vi "Calculate Saccade Gain.vi"(6 "Gain Window":T1, 7 "Impulse Data":refnum<data-value>, 8 "error in (no error)":errorcluster, 9 "Sample Rate (Hz)":dbl, 10 "Valid Range Fraction":dbl=1.0 format="%#_13g", 11 "Saccades in":T2[](array[typedef])) -> (0 "error out":errorcluster, 3 "Saccade out":T2[](array[typedef]))   [LabVIEW 2016]
uses:
  Saccade Analyser Saccade Data.ctl
  Saccade Analyser Impulse Data.ctl
  <vilib>/Analysis/NI_AALBase.lvlib
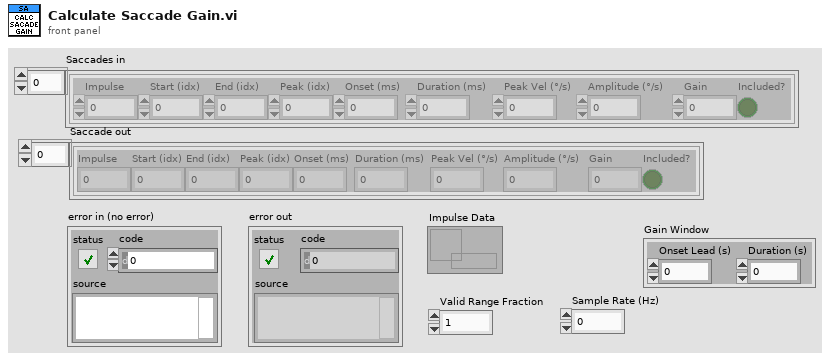
[diagram p1: front panel]
types:
  T1 = cluster{"Onset Lead (s)":dbl, "Duration (s)":dbl}
  T2 = typedef "Saccade Analyser Saccade Data.ctl" = cluster{"Impulse":i32, "Start (idx)":dbl, "End (idx)":dbl, "Peak (idx)":dbl, "Onset (ms)":dbl, "Duration (ms)":dbl, "Peak Vel (°/s)":dbl, "Amplitude (°/s)":dbl, "Gain":dbl, "Included?":bool}
  T3 = typedef "Saccade Analyser Impulse Data.ctl" = cluster{"Stimulus Data":dbl[], "Response Data":dbl[], "Peak (idx)":i32, "Onset (idx)":i32}
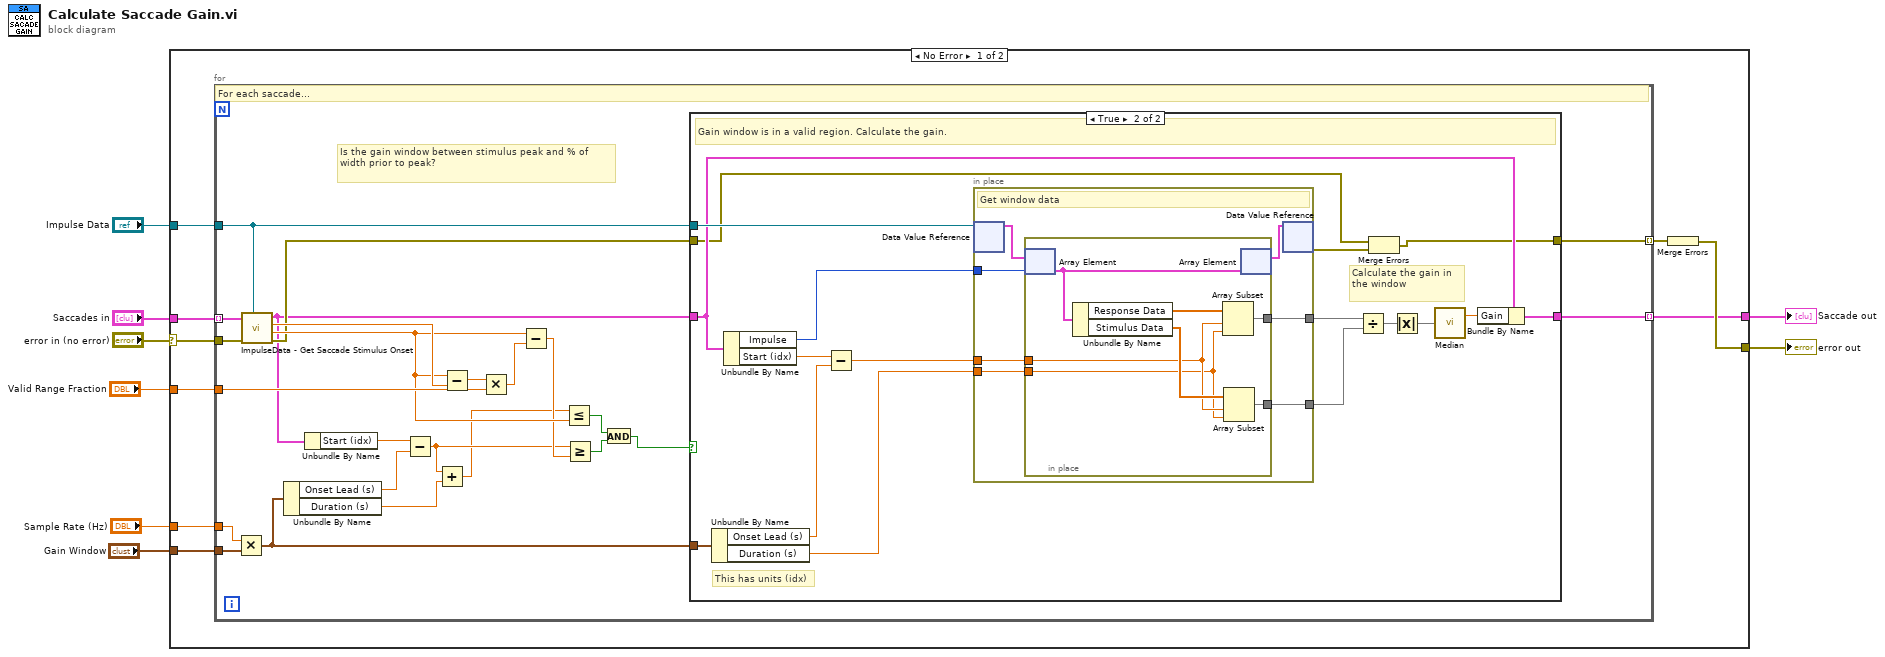
[diagram p0: block diagram]
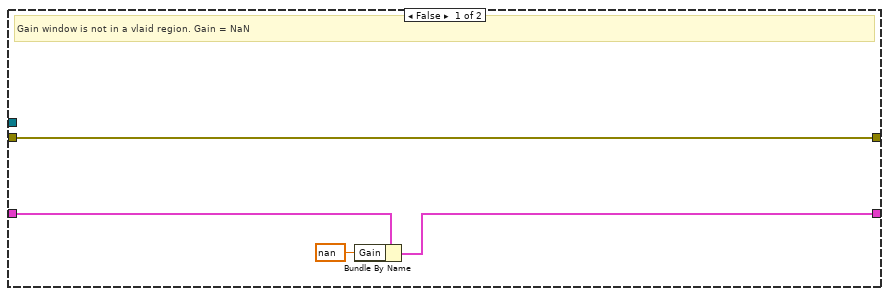
[diagram p2: hidden frame]
diagram:
  n1 = case shown="No Error" "error in (no error)" {
    selector: "error in (no error)" -> [w15 w77]
    tunnel: "Saccades in" -> [w17 w78]
    tunnel: [w12 w78] -> w5
    tunnel: [w14 w77] -> w7
    tunnel: "Impulse Data" -> [w16 _]
    tunnel: "Sample Rate (Hz)" -> [w13 _]
    tunnel: "Gain Window" -> [w11 _]
    tunnel: "Valid Range Fraction" -> [w10 _]
    frame No Error {
      n2 = for {
        tunnel: w17 -> [w38] mode=indexing
        tunnel: w16 -> [w36]
        tunnel: w15 -> [w37]
        tunnel: w13 -> [w40]
        tunnel: [w39] -> w12 mode=indexing
        tunnel: w11 -> [w41]
        tunnel: w10 -> [w33]
        tunnel: [w28] -> w9 mode=indexing
        # "Is the gain window between stimulus peak and % of width prior to peak?"
        # "For each saccade..."
        n3 = Multiply(x=w40, y=w41) -> (x*y=w25:T1)
        n4 = call "ImpulseData - Get Saccade Stimulus Onset.vi"("Saccade in"=w38, "error in (no error)"=w37, "Impulse Data"=w36) -> ("Saccade out"=w27:T2, "Onset (idx)"=w35:dbl, "Peak (idx)"=w32:dbl, "error out"=w29:errorcluster)  [unwired: 4 in]
        n5 = Unbundle By Name(w25) -> ("Onset Lead (s)"=w24:dbl, "Duration (s)"=w23:dbl)
        n6 = Unbundle By Name(w27) -> ("Start (idx)"=w26:dbl)
        n7 = Subtract(x=w26, y=w24) -> (x-y=w22:dbl)
        n8 = Add(x=w22, y=w23) -> (x+y=w21:dbl)
        n9 = Subtract(x=w32, y=w35) -> (x-y=w34:dbl)
        n10 = Multiply(x=w34, y=w33) -> (x*y=w31:dbl)
        n11 = Subtract(x=w32, y=w31) -> (x-y=w30:dbl)
        n12 = Less Or Equal?(x=w21, y=w32) -> (x <= y?=w20:bool)
        n13 = Greater Or Equal?(x=w22, y=w30) -> (x >= y?=w19:bool)
        n14 = And(x=w20, y=w19) -> (x .and. y?=w18:bool)
        n15 = case shown="True" w18 {
          tunnel: [w44 w59] -> w39
          tunnel: w36 -> [_ w56]
          tunnel: w27 -> [w45 w54]
          tunnel: w25 -> [_ w53]
          tunnel: w29 -> [w42 w47]
          tunnel: [w42 w46] -> w28
          frame False {
            # "Gain window is not in a vlaid region. Gain = NaN"
            n16 = Bundle By Name(cluster=w45, "Gain"=nan) -> (w44:T2)
          }
          frame True {
            # "This has units (idx)"
            # "Calculate the gain in the window"
            # "Gain window is in a valid region. Calculate the gain."
            n17 = Unbundle By Name(w53) -> ("Onset Lead (s)"=w51:dbl, "Duration (s)"=w49:dbl)
            n18 = Unbundle By Name(w54) -> ("Impulse"=w55:i32, "Start (idx)"=w52:dbl)
            n19 = Subtract(x=w52, y=w51) -> (x-y=w50:dbl)
            n20 = in-place {
              in-place-border: w55 -> [w67]
              in-place-border: w50 -> [w66]
              in-place-border: w49 -> [w65]
              in-place-border: [w64] -> w57
              in-place-border: [w63] -> w58
              # "Get window data"
              n21 = in-place-dvr #1(w56) -> (w69:T3[])  [unwired: 1 out]
              n22 = in-place {
                in-place-border: w66 -> [w72]
                in-place-border: w65 -> [w71]
                in-place-border: [w74] -> w64
                in-place-border: [w70] -> w63
                n23 = in-place-array #2(w69, w67) -> (w76:T3)
                n24 = Unbundle By Name(w76) -> ("Response Data"=w75:dbl[], "Stimulus Data"=w73:dbl[])
                n25 = Array Subset(array=w75, index=w72, length=w71) -> (w74:dbl[])
                n26 = Array Subset(array=w73, index=w72, length=w71) -> (w70:dbl[])
                n27 = in-place-array #2(w76) -> (w68:T3[])  [unwired: 1 out]
              }
              n28 = in-place-dvr #1(w68) -> (w48:errorcluster)  [unwired: 1 out]
            }
            n29 = Divide(x=w57, y=w58) -> (x/y=w62:dbl[])
            n30 = Merge Errors(w47, w48) -> (w46:errorcluster)
            n31 = Absolute Value(x=w62) -> (abs(x)=w61:dbl[])
            n32 = call <vilib>:"Median.vi"("X"=w61) -> ("median"=w60:dbl)  [unwired: 1 out]
            n33 = Bundle By Name(cluster=w54, "Gain"=w60) -> (w59:T2)
          }
        }
      }
      n34 = Merge Errors(w9) -> (w14:errorcluster)
    }
    frame Error {
    }
  }
  "error out" <- w7
  "Saccade out" <- w5
